vi "create_NG_folder.vi"(11 "output folder in":path) -> (3 "NG folder array":string[](array[string]))   [LabVIEW 2017]
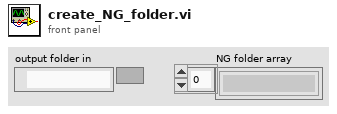
[diagram p1: front panel]
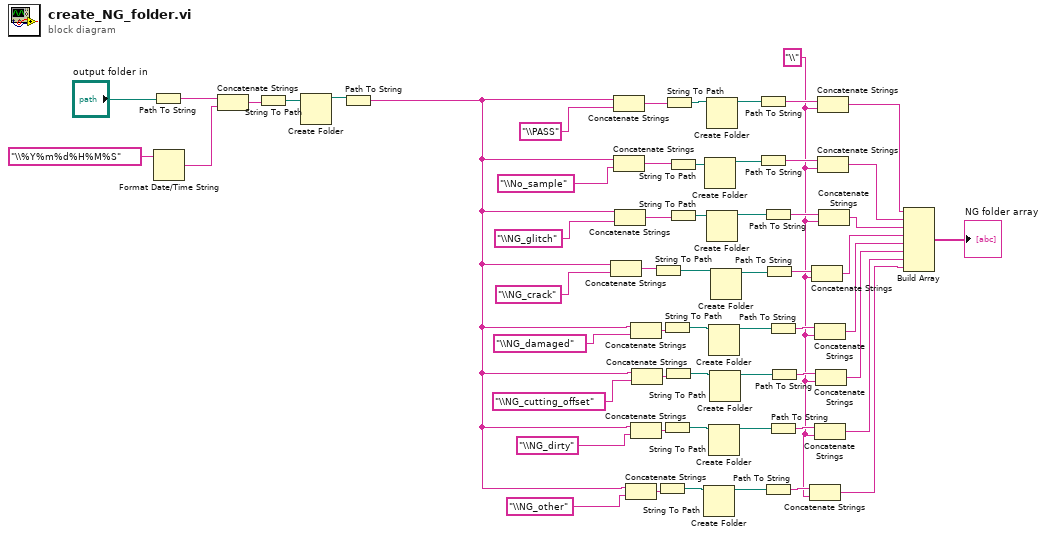
[diagram p0: block diagram]
diagram:
  w1 = "\\" ("string")
  n1 = Path To String(path="output folder in") -> (string=w32:string)
  n2 = Format Date/Time String(time format string (%c)="\\%Y%m%d%H%M%S") -> (date/time string=w31:string)  [unwired: 2 in]
  n3 = Concatenate Strings(w32, w31) -> (w30:string)
  n4 = String To Path(string=w30) -> (path=w29:path)
  n5 = Create Folder(path (use dialog)=w29) -> (created path=w28:path)  [unwired: 2 in, 2 out]
  n6 = Path To String(path=w28) -> (string=w3:string)
  n7 = Concatenate Strings(w3, "\\NG_crack" ("string")) -> (w53:string)
  n8 = Concatenate Strings(w3, "\\PASS" ("string")) -> (w49:string)
  n9 = Concatenate Strings(w3, "\\No_sample" ("string")) -> (w50:string)
  n10 = Concatenate Strings(w3, "\\NG_glitch" ("string")) -> (w52:string)
  n11 = Concatenate Strings(w3, "\\NG_other" ("string")) -> (w5:string)
  n12 = Concatenate Strings(w3, "\\NG_damaged" ("string")) -> (w54:string)
  n13 = Concatenate Strings(w3, "\\NG_dirty" ("string")) -> (w19:string)
  n14 = Concatenate Strings(w3, "\\NG_cutting_offset" ("string")) -> (w23:string)
  n15 = String To Path(string=w53) -> (path=w56:path)
  n16 = String To Path(string=w5) -> (path=w4:path)
  n17 = String To Path(string=w54) -> (path=w57:path)
  n18 = String To Path(string=w19) -> (path=w20:path)
  n19 = String To Path(string=w23) -> (path=w22:path)
  n20 = String To Path(string=w49) -> (path=w48:path)
  n21 = String To Path(string=w50) -> (path=w51:path)
  n22 = String To Path(string=w52) -> (path=w55:path)
  n23 = Create Folder(path (use dialog)=w4) -> (created path=w6:path)  [unwired: 2 in, 2 out]
  n24 = Create Folder(path (use dialog)=w51) -> (created path=w45:path)  [unwired: 2 in, 2 out]
  n25 = Create Folder(path (use dialog)=w48) -> (created path=w46:path)  [unwired: 2 in, 2 out]
  n26 = Create Folder(path (use dialog)=w55) -> (created path=w44:path)  [unwired: 2 in, 2 out]
  n27 = Create Folder(path (use dialog)=w57) -> (created path=w42:path)  [unwired: 2 in, 2 out]
  n28 = Create Folder(path (use dialog)=w20) -> (created path=w18:path)  [unwired: 2 in, 2 out]
  n29 = Create Folder(path (use dialog)=w22) -> (created path=w24:path)  [unwired: 2 in, 2 out]
  n30 = Create Folder(path (use dialog)=w56) -> (created path=w43:path)  [unwired: 2 in, 2 out]
  n31 = Path To String(path=w46) -> (string=w41:string)
  n32 = Path To String(path=w45) -> (string=w40:string)
  n33 = Path To String(path=w44) -> (string=w39:string)
  n34 = Path To String(path=w6) -> (string=w7:string)
  n35 = Path To String(path=w43) -> (string=w38:string)
  n36 = Path To String(path=w42) -> (string=w37:string)
  n37 = Path To String(path=w18) -> (string=w17:string)
  n38 = Path To String(path=w24) -> (string=w25:string)
  n39 = Concatenate Strings(w7, w1) -> (w2:string)
  n40 = Concatenate Strings(w38, w1) -> (w35:string)
  n41 = Concatenate Strings(w37, w1) -> (w34:string)
  n42 = Concatenate Strings(w17, w1) -> (w16:string)
  n43 = Concatenate Strings(w25, w1) -> (w21:string)
  n44 = Concatenate Strings(w41, w1) -> (w36:string)
  n45 = Concatenate Strings(w40, w1) -> (w27:string)
  n46 = Concatenate Strings(w39, w1) -> (w26:string)
  n47 = Build Array(w36, w27, w26, w35, w34, w21, w16, w2) -> (→"NG folder array":string[])
